vi "Consumer.vi"() -> ()   [LabVIEW 2011]
panel:
  out "element":string
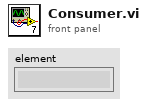
[diagram p1: front panel]
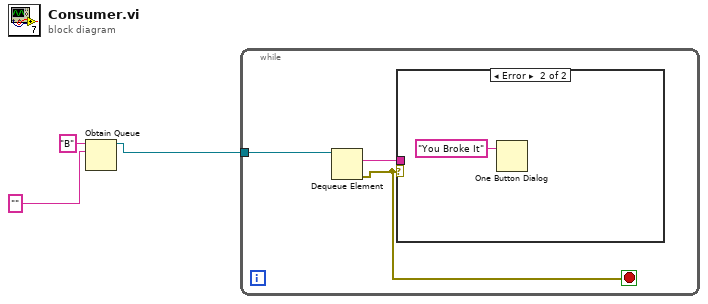
[diagram p0: block diagram]
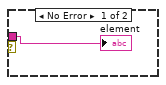
[diagram p2: hidden frame]
diagram:
  n1 = Obtain Queue(name (unnamed)="B", element data type="") -> (queue out=w1:refnum<queue>)  [unwired: 3 in, 2 out]
  n2 = while {
    tunnel: w1 -> [w6]
    stop <- w4 stop-if-true
    n3 = Dequeue Element(queue=w6) -> (element=w5:string, error out=w4:errorcluster)  [unwired: 2 in, 2 out]
    n4 = case shown="Error" w4 {
      tunnel: w5 -> [w7 _]
      frame No Error {
        "element" <- w7
      }
      frame Error {
        n5 = One Button Dialog(message="You Broke It") -> ()  [unwired: 1 in, 1 out]
      }
    }
  }
